vi "hmi_joe_johnson.vi"(11 "UserData":T1) -> ()   [LabVIEW 2011]
uses:
  user_data.ctl
  user_buttons_dualaction.ctl
  user_buttons_360.ctl
  joe_johnson/joe_johnson_state.ctl
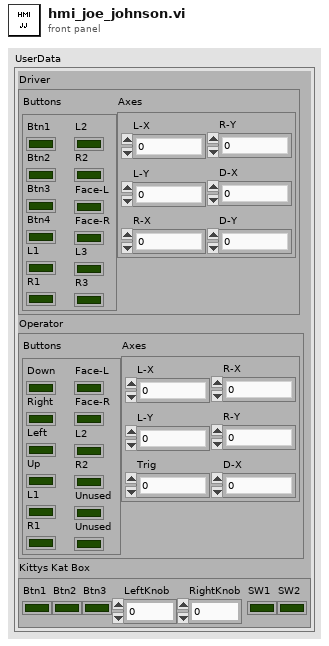
[diagram p1: front panel]
types:
  T1 = typedef "user_data.ctl" = cluster{"Driver":cluster{"Buttons":T2, "Axes":cluster{"L-X":dbl, "L-Y":dbl, "R-X":dbl, "R-Y":dbl, "D-X":dbl, "D-Y":dbl}}, "Operator":cluster{"Buttons":T3, "Axes":cluster{"L-X":dbl, "L-Y":dbl, "Trig":dbl, "R-X":dbl, "R-Y":dbl, "D-X":dbl}}, "Kittys Kat Box":cluster{"Btn1":bool, "Btn2":bool, "Btn3":bool, "LeftKnob":dbl, "RightKnob":dbl, "SW1":bool, "SW2":bool}}
  T2 = typedef "user_buttons_dualaction.ctl" = cluster{"Btn1":bool, "Btn2":bool, "Btn3":bool, "Btn4":bool, "L1":bool, "R1":bool, "L2":bool, "R2":bool, "Face-L":bool, "Face-R":bool, "L3":bool, "R3":bool}
  T3 = typedef "user_buttons_360.ctl" = cluster{"Down":bool, "Right":bool, "Left":bool, "Up":bool, "L1":bool, "R1":bool, "Face-L":bool, "Face-R":bool, "L2":bool, "R2":bool, "Unused":bool, "Unused":bool}
  T4 = typedef "joe_johnson_state.ctl" = enum16{"fold", "down", "up", "ramp", "bridge_lift", "manual", "ramp_stay"}
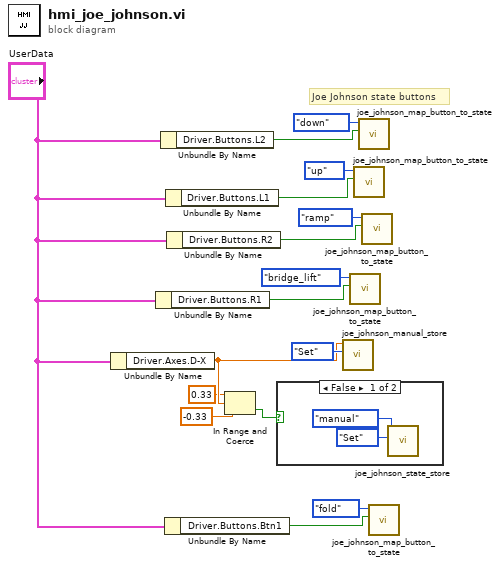
[diagram p0: block diagram]
diagram:
  # "Joe Johnson state buttons"
  n1 = Unbundle By Name("UserData") -> ("Driver.Axes.D-X"=w7:dbl)
  n2 = Unbundle By Name("UserData") -> ("Driver.Buttons.R1"=w9:bool)
  n3 = Unbundle By Name("UserData") -> ("Driver.Buttons.L2"=w14:bool)
  n4 = Unbundle By Name("UserData") -> ("Driver.Buttons.Btn1"=w3:bool)
  n5 = Unbundle By Name("UserData") -> ("Driver.Buttons.L1"=w15:bool)
  n6 = Unbundle By Name("UserData") -> ("Driver.Buttons.R2"=w16:bool)
  n7 = In Range and Coerce(upper limit=0.33, x=w7, lower limit=-0.33) -> (In Range?=w4:bool)  [unwired: 1 out]
  n8 = case shown="False" w4 {
    frame False {
      n9 = call "joe_johnson_state_store.vi"("data_store_mode"=enum16{"Set", "Get"}."Set", "joe_johnson_state"=joe_johnson_state."manual") -> ()  [unwired: 7 in, 3 out]
    }
    frame True {
    }
  }
  n10 = call "joe_johnson_manual_store.vi"("data_store_mode"=enum16{"Set", "Get"}."Set", "Man Command"=w7) -> ()  [unwired: 9 in, 1 out]
  n11 = call "joe_johnson_map_button_to_state.vi"("Button"=w9, "joe_johnson_state"=joe_johnson_state."bridge_lift") -> ()  [unwired: 10 in]
  n12 = call "joe_johnson_map_button_to_state.vi"("Button"=w15, "joe_johnson_state"=joe_johnson_state."up") -> ()  [unwired: 10 in]
  n13 = call "joe_johnson_map_button_to_state.vi"("Button"=w14, "joe_johnson_state"=joe_johnson_state."down") -> ()  [unwired: 10 in]
  n14 = call "joe_johnson_map_button_to_state.vi"("Button"=w16, "joe_johnson_state"=joe_johnson_state."ramp") -> ()  [unwired: 10 in]
  n15 = call "joe_johnson_map_button_to_state.vi"("Button"=w3, "joe_johnson_state"=joe_johnson_state."fold") -> ()  [unwired: 10 in]
